vi "Stimulus trigger logic-Live protocols.vi"(8 "Start trigger not fired":bool, 9 "Trigger lines value":T1, 10 "Tick Count(Ticks) in":u32, 11 "Trigger delays":T2={"Trigger period in live protocols (80MHz Cycles)"=510000000, "Pulse width in live protocols (80MHz Cycles)"=80000000, "Enable stimulus in live protocols"=FALSE, "Trigger delay in funct. protocols (80MHz Cycles)"=0, "Pulse width in funct. protocols (80MHz Cycles)"=400000, "Enable stimulus in funct. protocols"=FALSE}) -> (0 "Start trigger not fired":bool, 2 "Tick Count(Ticks) out":u32, 5 "Output value":bool)   [LabVIEW 2020]
uses:
  <vilib>/eio/EIONode/EIONode.xnode
  <vilib>/rvi/eio/common/nirviEmuTemplateMethod_errors.vi
  FPGA Typedefs/Stimulus trigger delays cluster.ctl
  FPGA Typedefs/PXI Trigger lines value cluster.ctl
panel:
  out "RAW counter VI":u32
  # "Limited to 53.5 sec (if U32)"
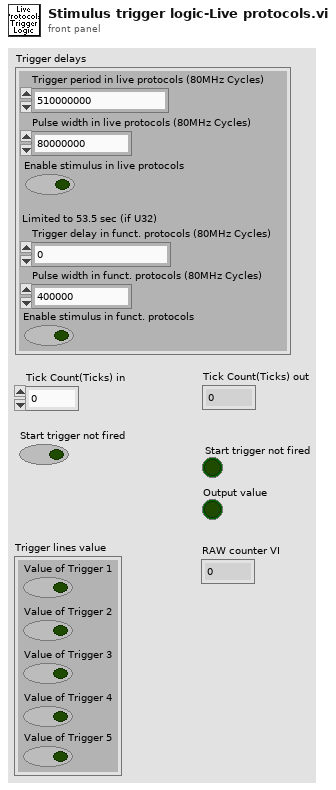
[diagram p1: front panel]
types:
  T1 = typedef "PXI Trigger lines value cluster.ctl" = cluster{"Value of Trigger 1":bool, "Value of Trigger 2":bool, "Value of Trigger 3":bool, "Value of Trigger 4":bool, "Value of Trigger 5":bool}
  T2 = typedef "Stimulus trigger delays cluster.ctl" = cluster{"Trigger period in live protocols (80MHz Cycles)":u32, "Pulse width in live protocols (80MHz Cycles)":u32, "Enable stimulus in live protocols":bool, "Trigger delay in funct. protocols (80MHz Cycles)":u32, "Pulse width in funct. protocols (80MHz Cycles)":u32, "Enable stimulus in funct. protocols":bool}
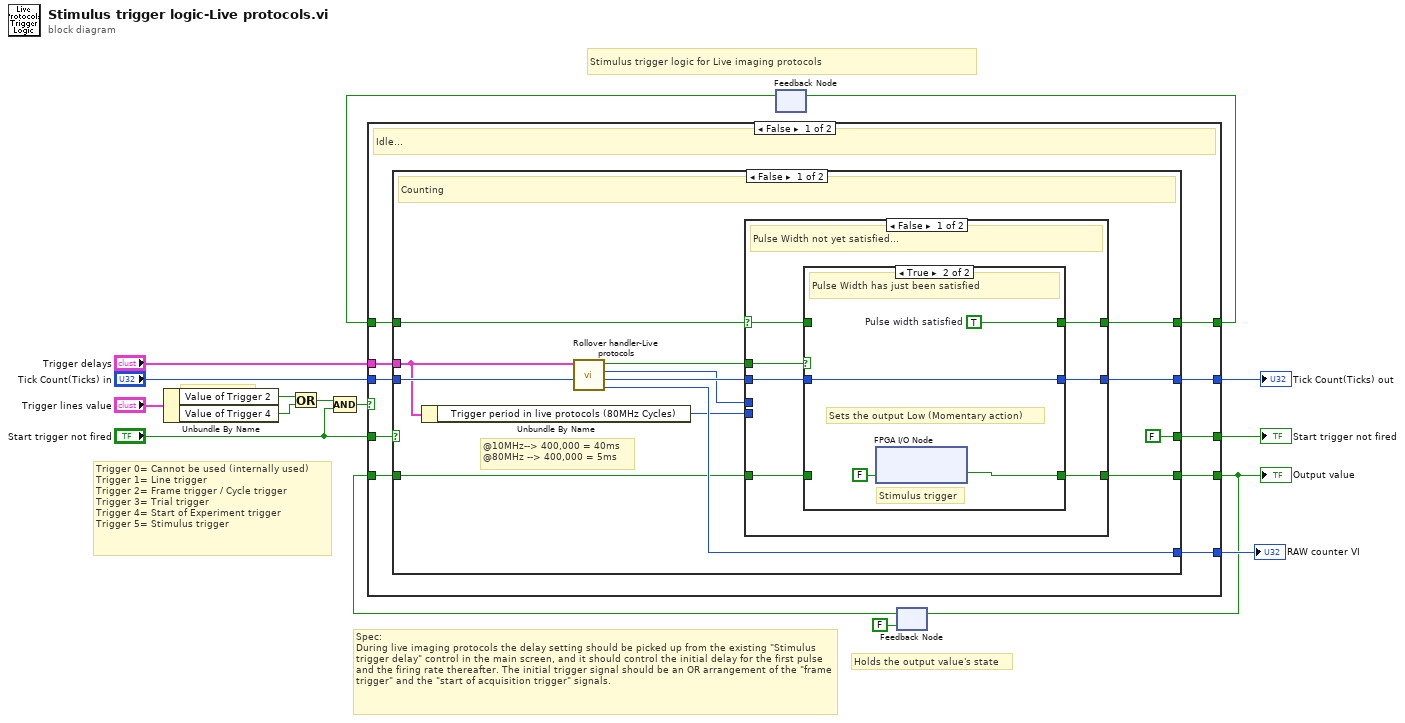
[diagram p0: block diagram]
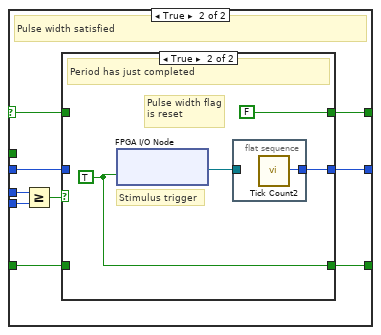
[diagram p3: hidden frame]
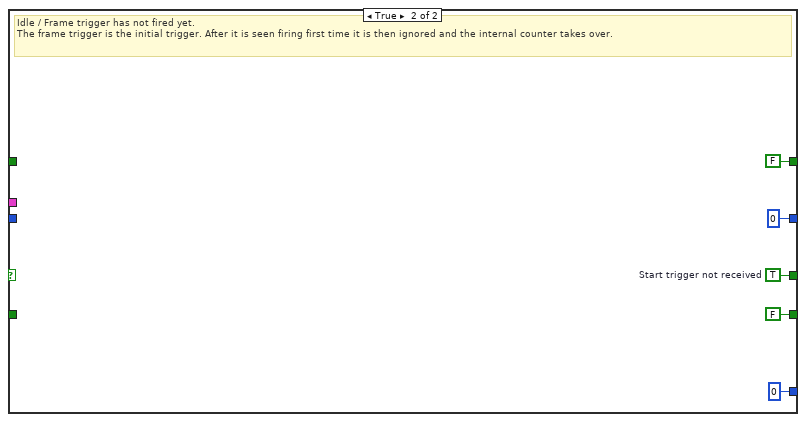
[diagram p5: hidden frame]
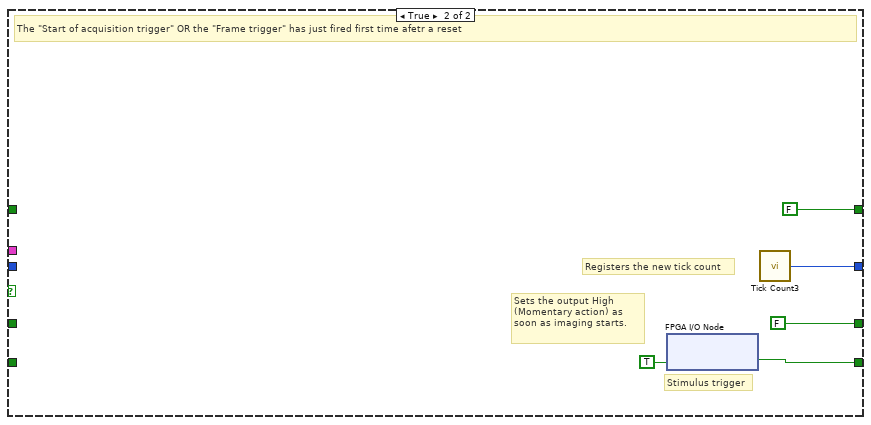
[diagram p6: hidden frame]
diagram:
  # "Holds the output value's state"
  # "Trigger 0= Cannot be used (internally used)\nTrigger 1= Line trigger\nTrigger 2= Frame trigger / Cycle trigger\nTrigger 3= Trial trigger\nTrigger 4= Start of Experiment trigger\nTrigger 5= Stimulus trigger"
  # "Frame trigger"
  # "Spec:\nDuring live imaging protocols the delay setting should be picked up from the existing \"Stimulus trigger delay\" control in the main screen, and it should control the initial delay for the first pulse and the firing rate thereafter. The initial trigger signal should be an OR arrangement of the \"frame trigger\" and the \"start of acquisition trigger\" signals."
  # "Stimulus trigger logic for Live imaging protocols"
  n1 = Unbundle By Name("Trigger lines value") -> ("Value of Trigger 2"=w9:bool, "Value of Trigger 4"=w7:bool)
  n2 = Or(x=w9, y=w7) -> (x .or. y?=w8:bool)
  n3 = Compound Arithmetic op=AND(w8, "Start trigger not fired") -> (w11:bool)
  n4 = feedback #1() -> (w1:bool)  [unwired: 1 in]
  n5 = feedback #2(FALSE ("PXI_Trig0")) -> (w3:bool)
  n6 = case shown="False" w11 {
    tunnel: [w24 w78] -> w12
    tunnel: "Tick Count(Ticks) in" -> [w26 _]
    tunnel: [w22 FALSE ("Reset")] -> w14
    tunnel: "Start trigger not fired" -> [w25 _]
    tunnel: "Trigger delays" -> [w23 _]
    tunnel: [w21 _] -> w6
    tunnel: [w20 w76] -> w4
    tunnel: w3 -> [w19 _]
    tunnel: [w18 FALSE ("Pulse width satisfied")] -> w2
    tunnel: w1 -> [w17 _]
    frame False {
      # "Idle..."
      n7 = case shown="False" w25 {
        tunnel: w26 -> [w36 _]
        tunnel: [w39 u32 0 ("Tick Count(Ticks)")] -> w24
        tunnel: w23 -> [w32 _]
        tunnel: [FALSE w71] -> w22
        tunnel: [w34 u32 0 ("Raw count")] -> w21
        tunnel: [w33 FALSE ("PXI_Trig0")] -> w20
        tunnel: w19 -> [w29 _]
        tunnel: [w28 FALSE ("Pulse width satisfied")] -> w18
        tunnel: w17 -> [w27 _]
        frame False {
          # "@10MHz--> 400,000 = 40ms\n@80MHz --> 400,000 = 5ms"
          # "Counting"
          n8 = Unbundle By Name(w32) -> ("Trigger period in live protocols (80MHz Cycles)"=w30:u32)
          n9 = call "Rollover handler-Live protocols.vi"("Tick Count Register in"=w36, "Trigger delays"=w32) -> ("Raw count"=w34:u32, "Tick Count Register out"=w35:u32, "Elapsed ticks count"=w31:u32, "Target reached"=w37:bool)  [unwired: 6 in]
          n10 = case shown="False" w27 {
            selector: w27 -> [w40 w56]
            tunnel: [w46 w58] -> w39
            tunnel: w29 -> [w45 w53]
            tunnel: w37 -> [w44 _]
            tunnel: w35 -> [w43 w55]
            tunnel: [w42 w54] -> w33
            tunnel: [w41 w57] -> w28
            tunnel: w30 -> [_ w61]
            tunnel: w31 -> [_ w60]
            frame False {
              # "Pulse Width not yet satisfied..."
              n11 = case shown="True" w44 {
                tunnel: w43 -> [w49 w51]
                tunnel: [w49 w51] -> w46
                tunnel: [w48 w52] -> w42
                tunnel: w45 -> [w48 _]
                tunnel: [w47 w50] -> w41
                tunnel: w40 -> [w47 _]
                frame False {
                  # "Pulse width not satisfied yet..."
                }
                frame True {
                  w50 = TRUE  # Pulse width satisfied
                  w52 = FALSE ("PXI_Trig0")
                  # "Sets the output Low (Momentary action)"
                  # "Stimulus trigger"
                  # "Pulse Width has just been satisfied"
                  n12 = xnode "FPGA I/O Node"("PXI_Trig5"=w52) -> ()  [unwired: 1 in, 1 out]
                }
              }
            }
            frame True {
              # "Pulse width satisfied"
              n13 = Greater Or Equal?(x=w60, y=w61) -> (x >= y?=w59:bool)
              n14 = case shown="True" w59 {
                tunnel: [w63 w67] -> w58
                tunnel: [w64 FALSE ("Pulse width satisfied")] -> w57
                tunnel: w56 -> [w64 _]
                tunnel: w55 -> [w63 _]
                tunnel: [w62 w65] -> w54
                tunnel: w53 -> [w62 _]
                frame False {
                  # "Period not completed yet..."
                }
                frame True {
                  w65 = TRUE ("PXI_Trig0")
                  # "Pulse width flag is reset"
                  # "Stimulus trigger"
                  # "Period has just completed"
                  n15 = xnode "FPGA I/O Node"("PXI_Trig5"=w65) -> ("FPGA I/O Out"=w68:refnum<k21>)  [unwired: 1 in]
                  n16 = flat-sequence {
                    tunnel: [w69] -> w67
                    tunnel: w68 -> [_]
                    frame #0 {
                      n17 = call "Tick Count2"() -> ("Tick Count(Ticks)"=w69:u32)
                    }
                  }
                }
              }
            }
          }
        }
        frame True {
          w71 = TRUE  # Start trigger not received
          # "Idle / Frame trigger has not fired yet. \nThe frame trigger is the initial trigger. After it is seen firing first time it is then ignored and the internal counter takes over."
        }
      }
    }
    frame True {
      w76 = TRUE ("PXI_Trig0")
      # "Registers the new tick count"
      # "Sets the output High (Momentary action) as soon as imaging starts."
      # "Stimulus trigger"
      # "The \"Start of acquisition trigger\" OR the \"Frame trigger\" has just fired first time afetr a reset"
      n18 = xnode "FPGA I/O Node"("PXI_Trig5"=w76) -> ()  [unwired: 1 in, 1 out]
      n19 = call "Tick Count3"() -> ("Tick Count(Ticks)"=w78:u32)
    }
  }
  "Start trigger not fired" <- w14
  "Tick Count(Ticks) out" <- w12
  "RAW counter VI" <- w6
  "Output value" <- w4
  n20 = feedback-in #1(w2) -> ()
  n21 = feedback-in #2(w4) -> ()
